vi "Image Zoom-in cleaned.vi"(8 "error in (no error)":errorcluster, 10 "Original":T2, 11 "Processed":T2) -> (0 "error out":errorcluster, 3 "Processed out":T2)   [LabVIEW 2011]
uses:
  <vilib>/vision/Image Controls.llb/IMAQ Image.ctl
  <vilib>/vision/NI_Vision_Development_Module.lvlib
panel:
  out "32bit integer":i32[](array[numeric])
  in  "input cluster":T1
  out "Array 2":cluster{i32, i32}[](array[cluster])
  out "Array":cluster{i32, i32}[](array[cluster])
  out "Original":T2(plugin-control)
  out "Processed":T2(plugin-control)
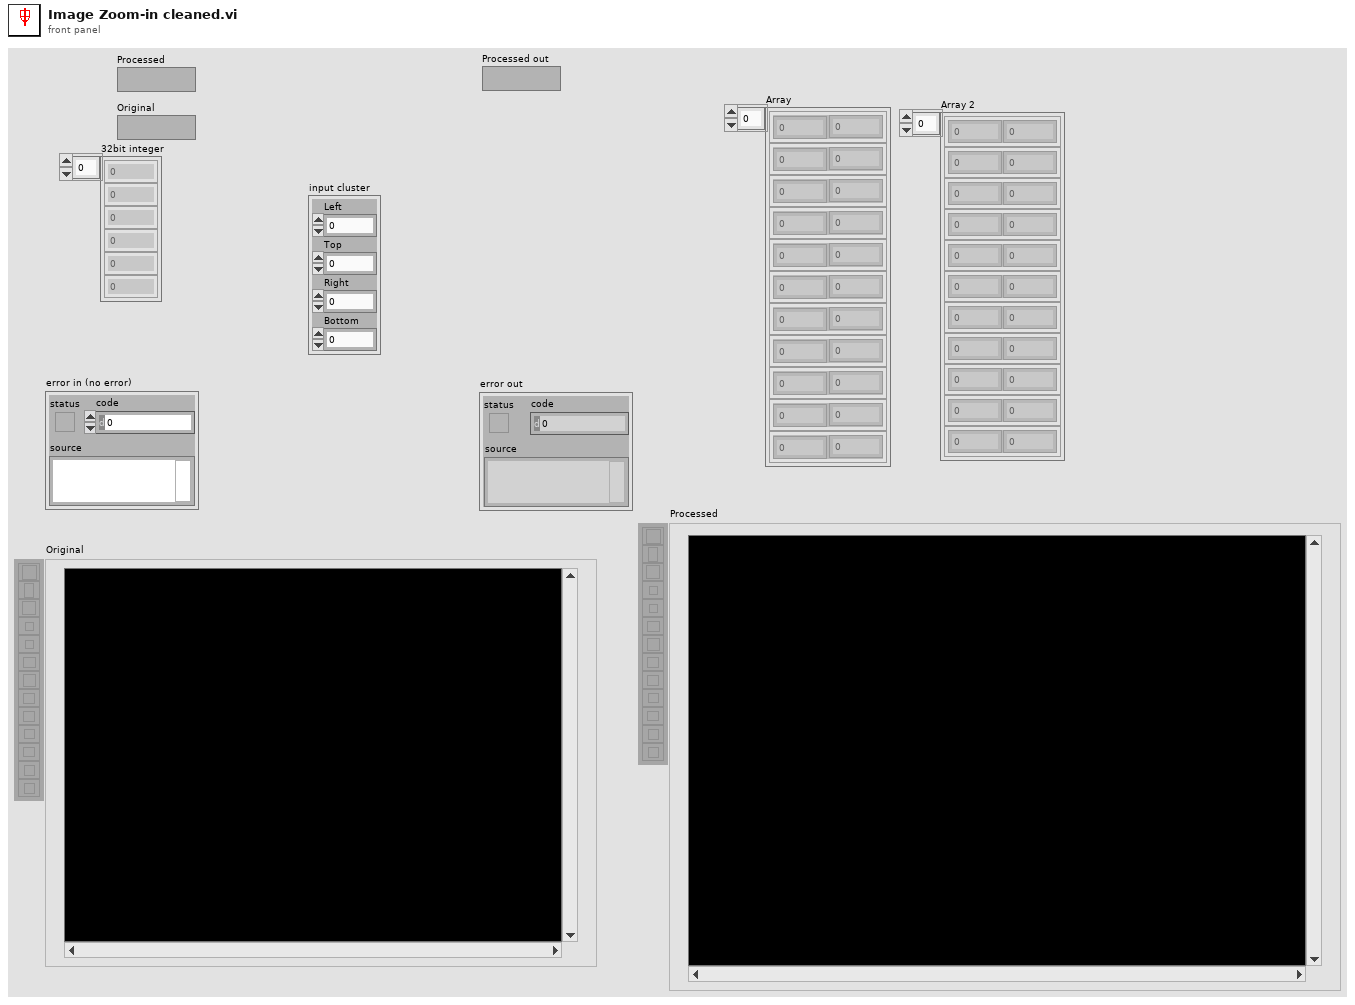
[diagram p1: front panel]
types:
  T1 = cluster{"Left":dbl, "Top":dbl, "Right":dbl, "Bottom":dbl}
  T2 = typedef "IMAQ Image.ctl" = refnum<image>
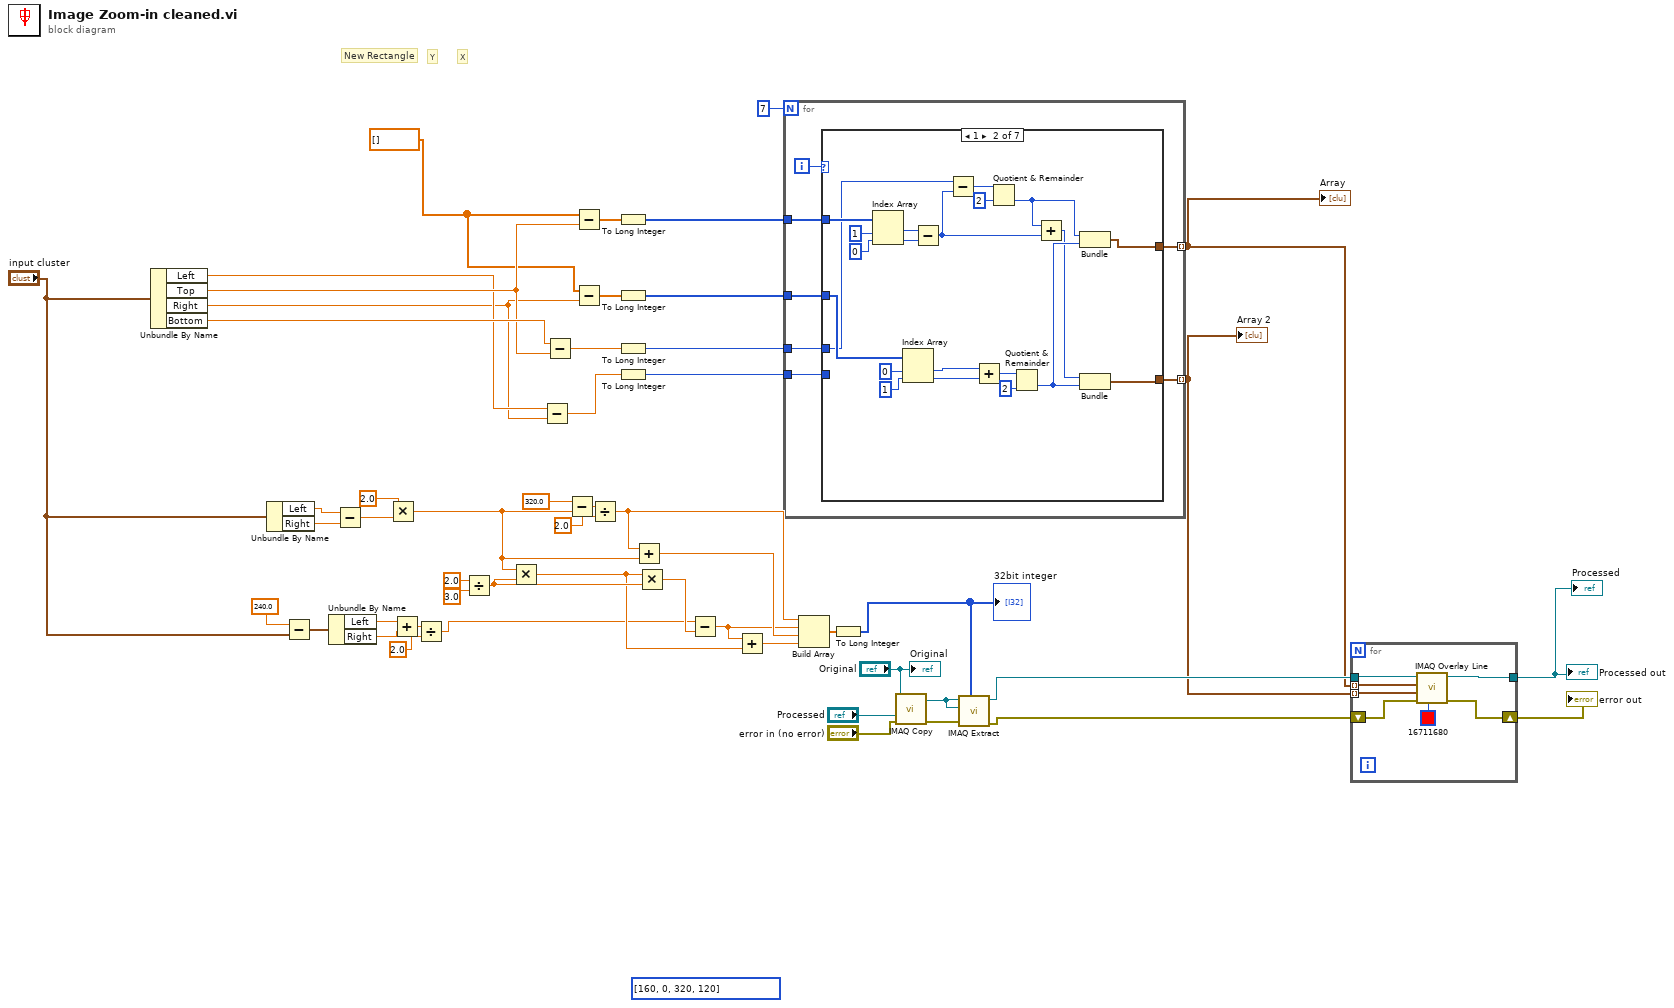
[diagram p0: block diagram]
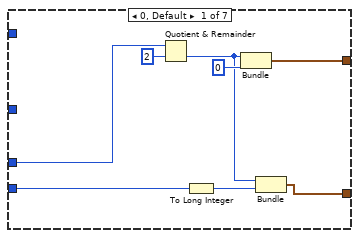
[diagram p2: hidden frame]
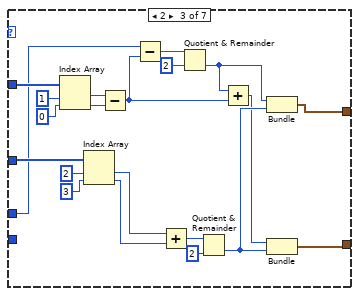
[diagram p3: hidden frame]
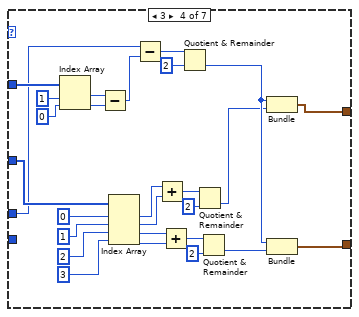
[diagram p4: hidden frame]
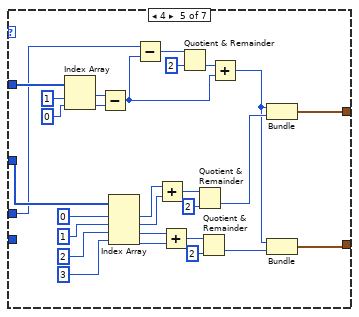
[diagram p5: hidden frame]
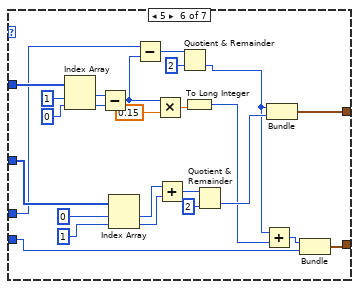
[diagram p6: hidden frame]
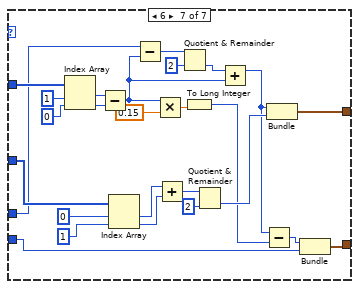
[diagram p7: hidden frame]
diagram:
  w28 = dbl[] []
  (unwired) i32[] [160, 0, 320, 120] ("Optional Rectangle")
  # "Y"
  # "X"
  # "New Rectangle"
  n1 = Unbundle By Name("input cluster") -> ("Left"=w38:dbl, "Top"=w40:dbl, "Right"=w37:dbl, "Bottom"=w41:dbl)
  n2 = Unbundle By Name("input cluster") -> ("Left"=w5:dbl, "Right"=w4:dbl)
  n3 = Subtract(x=240.0, y="input cluster") -> (x-y=w7:T1)
  n4 = Unbundle By Name(w7) -> ("Left"=w3:dbl, "Right"=w2:dbl)
  n5 = Subtract(x=w5, y=w4) -> (x-y=w27:dbl)
  n6 = Multiply(x=2.0, y=w27) -> (x*y=w15:dbl)
  n7 = Add(x=w3, y=w2) -> (x+y=w22:dbl)
  n8 = Divide(x=w22, y=2.0) -> (x/y=w9:dbl)
  n9 = Divide(x=2.0, y=3.0) -> (x/y=w18:dbl)
  n10 = Multiply(x=w15, y=w18) -> (x*y=w12:dbl)
  n11 = Subtract(x=w38, y=w37) -> (x-y=w36:dbl)
  n12 = Subtract(x=w41, y=w40) -> (x-y=w39:dbl)
  n13 = Subtract(x=320.0, y=w15) -> (x-y=w24:dbl)
  n14 = Subtract(x=w28, y=w40) -> (x-y=w32:dbl[])
  n15 = Subtract(x=w28, y=w37) -> (x-y=w31:dbl[])
  n16 = Divide(x=w24, y=2.0) -> (x/y=w16:dbl)
  n17 = To Long Integer(number=w32) -> (32bit integer=w30:i32[])
  n18 = To Long Integer(number=w31) -> (32bit integer=w29:i32[])
  n19 = To Long Integer(number=w39) -> (32bit integer=w35:i32)
  n20 = To Long Integer(number=w36) -> (32bit integer=w34:i32)
  n21 = Add(x=w16, y=w15) -> (x+y=w14:dbl)
  n22 = Multiply(x=w12, y=w18) -> (x*y=w17:dbl)
  n23 = Subtract(x=w9, y=w17) -> (x-y=w13:dbl)
  n24 = Add(x=w13, y=w12) -> (x+y=w11:dbl)
  n25 = for {
    N: 7 -> [_]
    tunnel: w30 -> [w56]
    tunnel: w29 -> [w55]
    tunnel: w35 -> [w58]
    tunnel: w34 -> [w57]
    tunnel: [w54] -> w43 mode=indexing
    tunnel: [w53] -> w42 mode=indexing
    i -> [w59]
    n26 = case shown="1" w59 {
      tunnel: w58 -> [w61 w70 w91 w119 w147 w179 w205]
      tunnel: w57 -> [w67 _ _ _ _ w171 w197]
      tunnel: w56 -> [_ w86 w107 w134 w162 w187 w213]
      tunnel: w55 -> [_ w83 w104 w131 w159 w186 w212]
      tunnel: [w64 w82 w103 w130 w158 w185 w211] -> w54
      tunnel: [w63 w81 w102 w129 w157 w184 w210] -> w53
      frame 0, Default {
        n27 = Quotient & Remainder(x=w61, y=2) -> (floor(x/y)=w60:i32)  [unwired: 1 out]
        n28 = To Long Integer(number=w67) -> (32bit integer=w65:i32)
        n29 = Bundle(w60, 0) -> (w64:cluster{i32, i32})  [unwired: 1 in]
        n30 = Bundle(w60, w65) -> (w63:cluster{i32, i32})  [unwired: 1 in]
      }
      frame 1 {
        n31 = Index Array(array=w86, index #1=1 ("index"), index #2=0 ("index")) -> (element #1=w73:i32, element #2=w72:i32)
        n32 = Index Array(array=w83, index #1=0 ("index"), index #2=1 ("index")) -> (element #1=w80:i32, element #2=w79:i32)
        n33 = Subtract(x=w73, y=w72) -> (x-y=w69:i32)
        n34 = Subtract(x=w70, y=w69) -> (x-y=w71:i32)
        n35 = Add(x=w80, y=w79) -> (x+y=w78:i32)
        n36 = Quotient & Remainder(x=w71, y=2) -> (floor(x/y)=w68:i32)  [unwired: 1 out]
        n37 = Quotient & Remainder(x=w78, y=2) -> (floor(x/y)=w76:i32)  [unwired: 1 out]
        n38 = Add(x=w68, y=w69) -> (x+y=w74:i32)
        n39 = Bundle(w68, w76) -> (w82:cluster{i32, i32})  [unwired: 1 in]
        n40 = Bundle(w74, w76) -> (w81:cluster{i32, i32})  [unwired: 1 in]
      }
      frame 2 {
        n41 = Index Array(array=w107, index #1=1 ("index"), index #2=0 ("index")) -> (element #1=w94:i32, element #2=w93:i32)
        n42 = Index Array(array=w104, index #1=2 ("index"), index #2=3 ("index")) -> (element #1=w101:i32, element #2=w100:i32)
        n43 = Subtract(x=w94, y=w93) -> (x-y=w90:i32)
        n44 = Subtract(x=w91, y=w90) -> (x-y=w92:i32)
        n45 = Add(x=w101, y=w100) -> (x+y=w99:i32)
        n46 = Quotient & Remainder(x=w92, y=2) -> (floor(x/y)=w89:i32)  [unwired: 1 out]
        n47 = Quotient & Remainder(x=w99, y=2) -> (floor(x/y)=w97:i32)  [unwired: 1 out]
        n48 = Add(x=w89, y=w90) -> (x+y=w95:i32)
        n49 = Bundle(w89, w97) -> (w103:cluster{i32, i32})  [unwired: 1 in]
        n50 = Bundle(w95, w97) -> (w102:cluster{i32, i32})  [unwired: 1 in]
      }
      frame 3 {
        n51 = Index Array(array=w134, index #1=1 ("index"), index #2=0 ("index")) -> (element #1=w122:i32, element #2=w121:i32)
        n52 = Subtract(x=w122, y=w121) -> (x-y=w118:i32)
        n53 = Index Array(array=w131, index #1=0 ("index"), index #2=1 ("index"), index #3=2 ("index"), index #4=3 ("index")) -> (element #1=w112:i32, element #2=w111:i32, element #3=w128:i32, element #4=w127:i32)
        n54 = Subtract(x=w119, y=w118) -> (x-y=w120:i32)
        n55 = Add(x=w112, y=w111) -> (x+y=w113:i32)
        n56 = Add(x=w128, y=w127) -> (x+y=w126:i32)
        n57 = Quotient & Remainder(x=w120, y=2) -> (floor(x/y)=w117:i32)  [unwired: 1 out]
        n58 = Quotient & Remainder(x=w113, y=2) -> (floor(x/y)=w110:i32)  [unwired: 1 out]
        n59 = Quotient & Remainder(x=w126, y=2) -> (floor(x/y)=w124:i32)  [unwired: 1 out]
        n60 = Bundle(w117, w110) -> (w130:cluster{i32, i32})  [unwired: 1 in]
        n61 = Bundle(w117, w124) -> (w129:cluster{i32, i32})  [unwired: 1 in]
      }
      frame 4 {
        n62 = Index Array(array=w162, index #1=1 ("index"), index #2=0 ("index")) -> (element #1=w150:i32, element #2=w149:i32)
        n63 = Subtract(x=w150, y=w149) -> (x-y=w138:i32)
        n64 = Index Array(array=w159, index #1=0 ("index"), index #2=1 ("index"), index #3=2 ("index"), index #4=3 ("index")) -> (element #1=w141:i32, element #2=w140:i32, element #3=w156:i32, element #4=w155:i32)
        n65 = Subtract(x=w147, y=w138) -> (x-y=w148:i32)
        n66 = Add(x=w141, y=w140) -> (x+y=w142:i32)
        n67 = Add(x=w156, y=w155) -> (x+y=w154:i32)
        n68 = Quotient & Remainder(x=w148, y=2) -> (floor(x/y)=w146:i32)  [unwired: 1 out]
        n69 = Quotient & Remainder(x=w142, y=2) -> (floor(x/y)=w139:i32)  [unwired: 1 out]
        n70 = Quotient & Remainder(x=w154, y=2) -> (floor(x/y)=w152:i32)  [unwired: 1 out]
        n71 = Add(x=w146, y=w138) -> (x+y=w137:i32)
        n72 = Bundle(w137, w139) -> (w158:cluster{i32, i32})  [unwired: 1 in]
        n73 = Bundle(w137, w152) -> (w157:cluster{i32, i32})  [unwired: 1 in]
      }
      frame 5 {
        n74 = Index Array(array=w187, index #1=1 ("index"), index #2=0 ("index")) -> (element #1=w182:i32, element #2=w181:i32)
        n75 = Subtract(x=w182, y=w181) -> (x-y=w168:i32)
        n76 = Index Array(array=w186, index #1=0 ("index"), index #2=1 ("index")) -> (element #1=w174:i32, element #2=w173:i32)
        n77 = Subtract(x=w179, y=w168) -> (x-y=w180:i32)
        n78 = Multiply(x=w168, y=0.15) -> (x*y=w166:dbl)
        n79 = Add(x=w174, y=w173) -> (x+y=w175:i32)
        n80 = Quotient & Remainder(x=w180, y=2) -> (floor(x/y)=w169:i32)  [unwired: 1 out]
        n81 = To Long Integer(number=w166) -> (32bit integer=w165:i32)
        n82 = Quotient & Remainder(x=w175, y=2) -> (floor(x/y)=w172:i32)  [unwired: 1 out]
        n83 = Add(x=w169, y=w165) -> (x+y=w170:i32)
        n84 = Bundle(w169, w172) -> (w185:cluster{i32, i32})  [unwired: 1 in]
        n85 = Bundle(w170, w171) -> (w184:cluster{i32, i32})  [unwired: 1 in]
      }
      frame 6 {
        n86 = Index Array(array=w213, index #1=1 ("index"), index #2=0 ("index")) -> (element #1=w208:i32, element #2=w207:i32)
        n87 = Subtract(x=w208, y=w207) -> (x-y=w190:i32)
        n88 = Index Array(array=w212, index #1=0 ("index"), index #2=1 ("index")) -> (element #1=w200:i32, element #2=w199:i32)
        n89 = Subtract(x=w205, y=w190) -> (x-y=w206:i32)
        n90 = Multiply(x=w190, y=0.15) -> (x*y=w193:dbl)
        n91 = Add(x=w200, y=w199) -> (x+y=w201:i32)
        n92 = Quotient & Remainder(x=w206, y=2) -> (floor(x/y)=w195:i32)  [unwired: 1 out]
        n93 = To Long Integer(number=w193) -> (32bit integer=w192:i32)
        n94 = Quotient & Remainder(x=w201, y=2) -> (floor(x/y)=w198:i32)  [unwired: 1 out]
        n95 = Add(x=w195, y=w190) -> (x+y=w191:i32)
        n96 = Subtract(x=w191, y=w192) -> (x-y=w196:i32)
        n97 = Bundle(w191, w198) -> (w211:cluster{i32, i32})  [unwired: 1 in]
        n98 = Bundle(w196, w197) -> (w210:cluster{i32, i32})  [unwired: 1 in]
      }
    }
  }
  "Array" <- w43
  "Array 2" <- w42
  n99 = Build Array(w16, w13, w14, w11) -> (w10:dbl[])
  n100 = To Long Integer(number=w10) -> (32bit integer=w1:i32[])
  "32bit integer" <- w1
  n101 = call "IMAQ Copy"("error in (no error)"="error in (no error)", "Image Dst"="Processed", "Image Src"="Original") -> ("error out"=w49:errorcluster, "Image Dst Out"=w51:T2)  [unwired: 3 in]
  n102 = call "IMAQ Extract"("Optional Rectangle"=w1, "error in (no error)"=w49, "Image Dst"=w51, "Image Src"=w51) -> ("error out"=w48:errorcluster, "Image Dst Out"=w52:T2)  [unwired: 6 in]
  n103 = for {
    tunnel: w52 -> [w221]
    tunnel: [w220] -> w46
    tunnel: w43 -> [w219] mode=indexing
    tunnel: w42 -> [w218] mode=indexing
    shift-right: [w216] -> w47
    shift-left: w48 -> [w217]
    n104 = call "IMAQ Overlay Line"("Color"=u32 16711680, "error in (no error)"=w217, "End Point"=w218, "Start Point"=w219, "Image"=w221) -> ("error out"=w216:errorcluster, "Image Out"=w220:T2)  [unwired: 5 in]
  }
  "Processed out" <- w46
  "error out" <- w47
  "Processed" <- w46
  "Original" <- "Original"
